vi "date_and_time.vi"() -> (0 "Date":string)   [LabVIEW 2024]
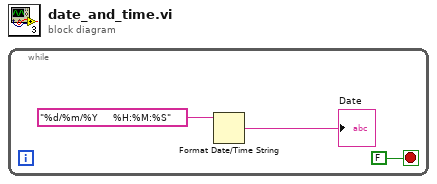
[diagram p0: block diagram]
diagram:
  n1 = while {
    stop <- FALSE stop-if-true
    n2 = Format Date/Time String(time format string (%c)="%d/%m/%Y     %H:%M:%S") -> (date/time string=→"Date":string)  [unwired: 2 in]
  }
